vi "Data Array to Cluster.vi"(11 "Data":dbl[](array[numeric])) -> (3 "Data out":T1(array[cluster]))   [LabVIEW 2022 SP3, in "Cryo Cooler.lvclass"]
uses:
  Cryo Cooler.lvclass
  Cryo Cooler.lvclass/Cryo Cooler.ctl
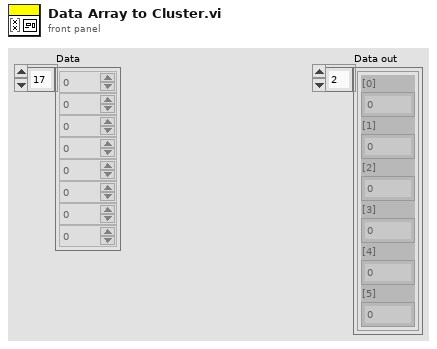
[diagram p1: front panel]
types:
  T1 = cluster{"[0]":dbl, "[1]":dbl, "[2]":dbl, "[3]":dbl, "[4]":dbl, "[5]":dbl}[]
  T2 = cluster{"[0]":dbl, "[1]":dbl, "[2]":dbl, "[3]":dbl, "[4]":dbl, "[5]":dbl}
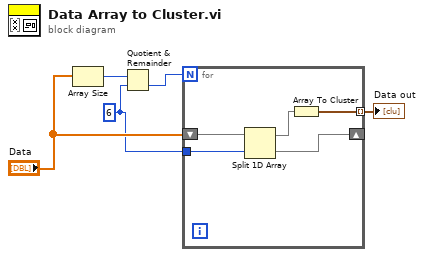
[diagram p0: block diagram]
diagram:
  w2 = 6 ("y")
  n1 = Array Size(array="Data") -> (size(s)=w5:i32)
  n2 = Quotient & Remainder(x=w5, y=w2) -> (floor(x/y)=w4:i32)  [unwired: 1 out]
  n3 = for {
    N: w4 -> [_]
    shift-right: [w6] -> _
    shift-left: "Data" -> [w10]
    tunnel: w2 -> [w9]
    tunnel: [w7] -> w1 mode=indexing
    n4 = Split 1D Array(array=w10, index=w9) -> (first subarray=w8:dbl[], second subarray=w6:dbl[])
    n5 = Array To Cluster(array=w8) -> (cluster=w7:T2)
  }
  "Data out" <- w1
